vi "Command Type.vi"(11 "Stop Seq Command Config in":refnum<class "Stop Seq Command Config.lvclass">) -> (2 "Command Type":string)   [LabVIEW 2020, in "VolatusSeqConfig.lvlib" / "Stop Seq Command Config.lvclass"]
uses:
  Stop Seq Command Config.lvclass
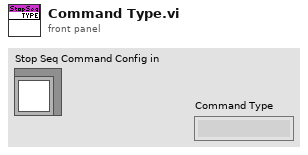
[diagram p1: front panel]
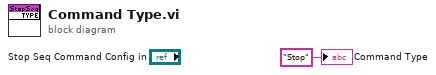
[diagram p0: block diagram]
diagram:
  "Command Type" <- "Stop" ("Command Type")
